vi "PPL Paths.vi"() -> (1 "Renamed PPL Path":path, 2 "PPL Path":path)   [LabVIEW 2020]
doc: "Returns the paths for the lv_icon.lvlibp file and its backup paths."
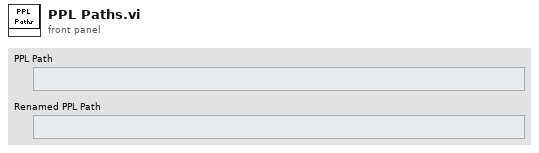
[diagram p1: front panel]
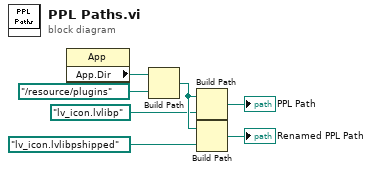
[diagram p0: block diagram]
diagram:
  n1 = property class="App"() -> ("App.Dir"=w1:path)  [unwired: 2 in, 2 out]
  n2 = Build Path(base path=w1, name or relative path=path "../resource/plugins" ("symbolic path")) -> (appended path=w7:path)
  n3 = Build Path(base path=w7, name or relative path=path "lv_icon.lvlibp") -> (appended path=→"PPL Path":path)
  n4 = Build Path(base path=w7, name or relative path=path "lv_icon.lvlibpshipped") -> (appended path=→"Renamed PPL Path":path)
